vi "Read Scan Position (Scan).vi"(8 "error in (no error)":errorcluster, 11 "VISA resource name":refnum<visa-resource-name>) -> (0 "error out":errorcluster, 2 "Scan Position":u16, 3 "VISA resource name out":refnum<visa-resource-name>)   [LabVIEW 2015, in "SRS SR400.lvlib"]
doc: "<B>NN</B>\n\nThe NN command reads the scan position. The scan position is the number of count periods or data points completed so far during the current scan and is shown in the brackets on the N PERIODS menu line. The NN command is a read only command."
uses:
  SRS SR400.lvlib
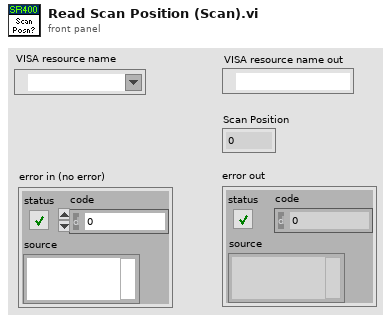
[diagram p1: front panel]
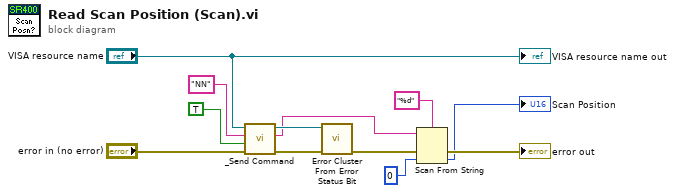
[diagram p0: block diagram]
diagram:
  n1 = call "_Send Command.vi"("error in (no error)"="error in (no error)", "Read Value? (F)"=TRUE, "Command"="NN" ("command"), "VISA resource name"="VISA resource name") -> ("error out"=w4:errorcluster, "Response"=w1:string, "VISA resource name out"=w3:refnum<visa-resource-name>)  [unwired: 5 out]
  n2 = call "Error Cluster From Error Status Bit.vi"("error in (no error)"=w4, "VISA resource name"=w3) -> ("error out"=w2:errorcluster)  [unwired: 8 in, 1 out]
  n3 = Scan From String(format string="%d", input string=w1, error in=w2, default 1=u16 0 ("default value 1")) -> (error out=→"error out":errorcluster, output 1=→"Scan Position":u16)  [unwired: 1 in, 2 out]
  "VISA resource name out" <- "VISA resource name"
